vi "Body Length Type.vi"(8 "error in (no error)":errorcluster, 11 "Request in":refnum<class "Request.lvclass">) -> (0 "error out":errorcluster, 2 "Body Length Type":T1, 3 "Request out":refnum<class "Request.lvclass">)   [LabVIEW 2020, in "HTTP Utils.lvlib" / "Request.lvclass"]
uses:
  Request.lvclass
  Body Length Type.ctl
  Request.lvclass/Request.ctl
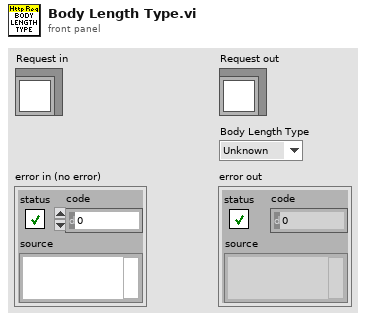
[diagram p1: front panel]
types:
  T1 = typedef "HTTP Utils.lvlib/Request.lvclass/Body Length Type.ctl" = enum16{"Unknown", "Length", "Chunked"}
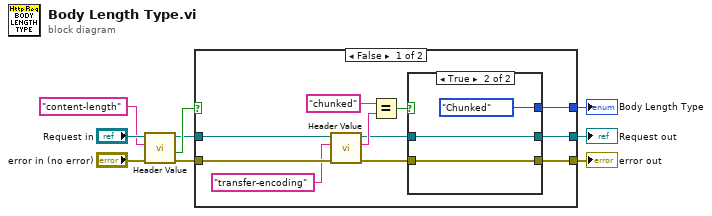
[diagram p0: block diagram]
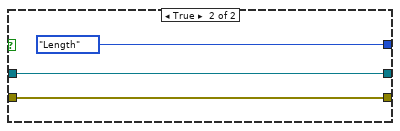
[diagram p3: hidden frame]
diagram:
  n1 = call "Header Value.vi"("error in (no error)"="error in (no error)", "Header"="content-length", "Request in"="Request in") -> ("error out"=w6:errorcluster, "Exists"=w5:bool, "Request out"=w4:refnum<class "Request.lvclass">)  [unwired: 5 in, 1 out]
  n2 = case shown="False" w5 {
    tunnel: w6 -> [w19 w27]
    tunnel: w4 -> [w20 w28]
    tunnel: [w12 w28] -> w3
    tunnel: [w11 w27] -> w2
    tunnel: [w10 Body_Length_Type."Length" ("Body Length")] -> w1
    frame False {
      n3 = call "Header Value.vi"("error in (no error)"=w19, "Header"="transfer-encoding", "Request in"=w20) -> ("error out"=w13:errorcluster, "Value"=w17:string, "Request out"=w14:refnum<class "Request.lvclass">)  [unwired: 5 in, 1 out]
      n4 = Equal?(x="chunked" ("Header"), y=w17) -> (x = y?=w15:bool)
      n5 = case shown="True" w15 {
        tunnel: w14 -> [w22 w25]
        tunnel: w13 -> [w21 w24]
        tunnel: [w22 w25] -> w12
        tunnel: [w21 w24] -> w11
        tunnel: [_ Body_Length_Type."Chunked" ("Body Length Type")] -> w10
        frame False {
        }
        frame True {
        }
      }
    }
    frame True {
    }
  }
  "error out" <- w2
  "Request out" <- w3
  "Body Length Type" <- w1
